vi "Get Header By Name.vi"(8 "error in (no error)":errorcluster, 10 "Name":string, 11 "Response Headers in":refnum<class "Response Headers.lvclass">) -> (0 "error out":errorcluster, 1 "Found?":bool, 2 "Value":string, 3 "Response Headers out":refnum<class "Response Headers.lvclass">)   [LabVIEW 2018, in "REST Client_JKI.lvlib" / "Response Headers.lvclass"]
doc: "Get a HTTP response header value by name.\n\nThe VI provides the following arguments.\n\n<b>Name</b> specifies the name of the HTTP header to get."
uses:
  Response Headers.lvclass
  Response Headers.lvclass/Response Headers.ctl
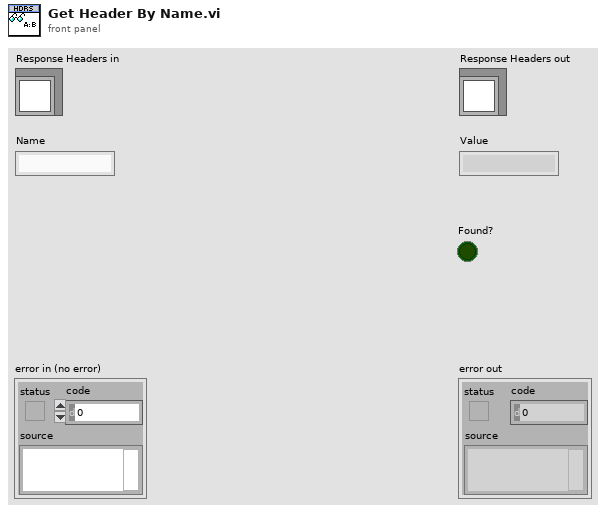
[diagram p1: front panel]
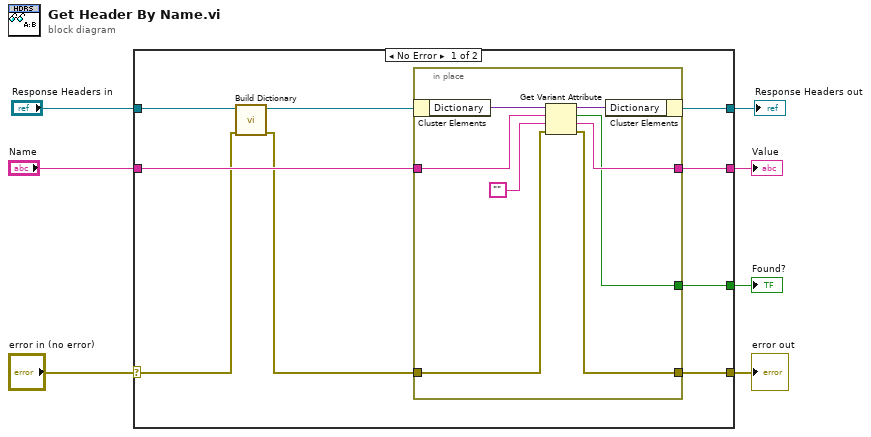
[diagram p0: block diagram]
diagram:
  n1 = case shown="No Error" "error in (no error)" {
    selector: "error in (no error)" -> [w9 w26]
    tunnel: [w14 w26] -> w6
    tunnel: [w16 w25] -> w4
    tunnel: "Response Headers in" -> [w11 w25]
    tunnel: "Name" -> [w15 _]
    tunnel: [w13 _] -> w2
    tunnel: [w12 _] -> w1
    frame No Error {
      n2 = call "Build Dictionary.vi"("error in (no error)"=w9, "Response Headers in"=w11) -> ("error out"=w8:errorcluster, "Response Headers out"=w10:refnum<class "Response Headers.lvclass">)  [unwired: 8 in]
      n3 = in-place {
        in-place-border: w15 -> [w22]
        in-place-border: w8 -> [w21]
        in-place-border: [w19] -> w14
        in-place-border: [w18] -> w13
        in-place-border: [w17] -> w12
        n4 = in-place-cluster #1(w10) -> ("Dictionary"=w24:variant)
        n5 = Get Variant Attribute(Variant=w24, name=w22, default value (empty Variant)="", error in=w21) -> (duplicate Variant=w23:variant, found=w17:bool, value=w18:string, error out=w19:errorcluster)
        n6 = in-place-cluster #1("Dictionary"=w23) -> (w16:refnum<class "Response Headers.lvclass">)
      }
    }
    frame Error {
    }
  }
  "error out" <- w6
  "Response Headers out" <- w4
  "Value" <- w2
  "Found?" <- w1
